vi "StackedSecuence_local.vi"() -> ()   [LabVIEW 2020]
panel:
  out "String 2":string
  in  "String":string
  out "Meter":dbl(knob) scale=0.0..10.0
  in  "Variador":dbl(knob) scale=0.0..10.0
  out "Boolean":bool
  in  "Interruptor":bool
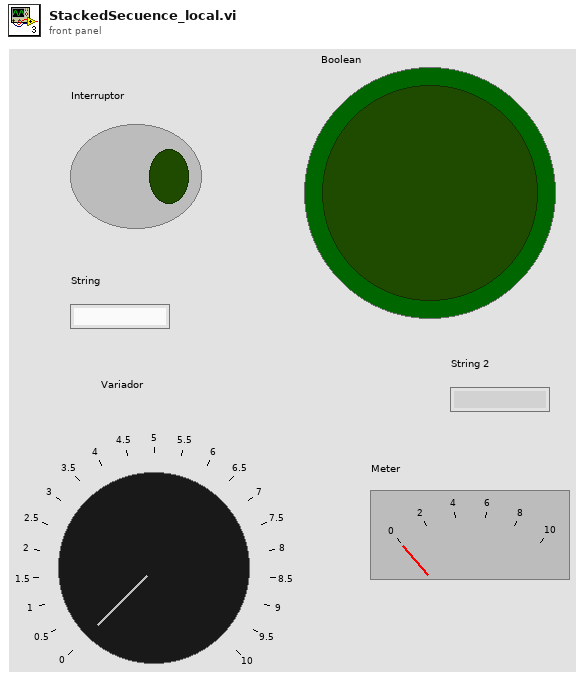
[diagram p1: front panel]
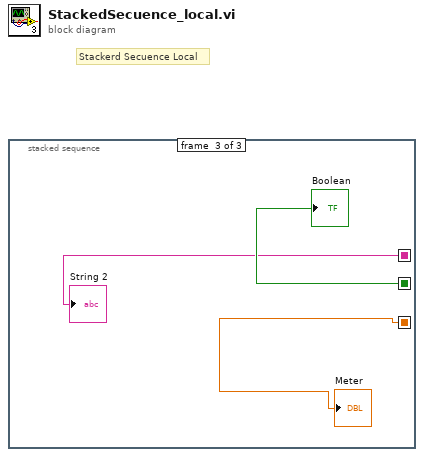
[diagram p0: block diagram]
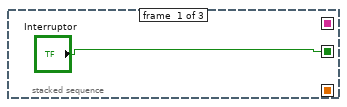
[diagram p2: hidden frame]
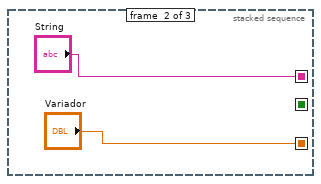
[diagram p3: hidden frame]
diagram:
  # "Stackerd Secuence Local"
  n1 = stacked-sequence {
    seq-local: ["Interruptor" _ _] -> [_ _ w6]
    seq-local: [_ "Variador" _] -> [_ _ w5]
    seq-local: [_ "String" _] -> [_ _ w4]
    frame #0 {
    }
    frame #1 {
    }
    frame #2 {
      "Boolean" <- w6
      "Meter" <- w5
      "String 2" <- w4
    }
  }
